vi "TestTracer.vi"() -> ()   [LabVIEW 2018]
uses:
  8343dff0-8b7c-4e66-97a3-4b21e463c662.vi
  7eb2ee23-5221-471e-a6d0-41069041a5d2.vi
  88696aa2-b6d8-4ac2-bba1-d74daa604035.vi
  a57bbf11-b234-4300-b227-3b603d238aca.vi
  ee03f129-e9c8-4ab2-bbd6-a9c7767b6f28.vi
  0673ade5-3870-4221-86d1-9f763805091c.vi
  TracerLibrary/Tracer/protected/SendMessage.vi
  TracerLibrary/Tracer/protected/Timestamp.vi
  TracerLibrary/Tracer/Tracer_Level-Debug.vi
  TracerLibrary/Tracer/protected/Tracer_ClassAttributes.vi
  TracerLibrary/Tracer/Tracer_Level-Warning.vi
  TracerLibrary/Tracer/Tracer_Level-Info.vi
  TracerLibrary/Tracer/Tracer_Level-Error.vi
  TracerLibrary/Tracer/Tracer.lvclass
panel:
  out "Ms / Tracecall":dbl
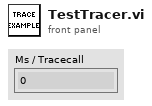
[diagram p1: front panel]
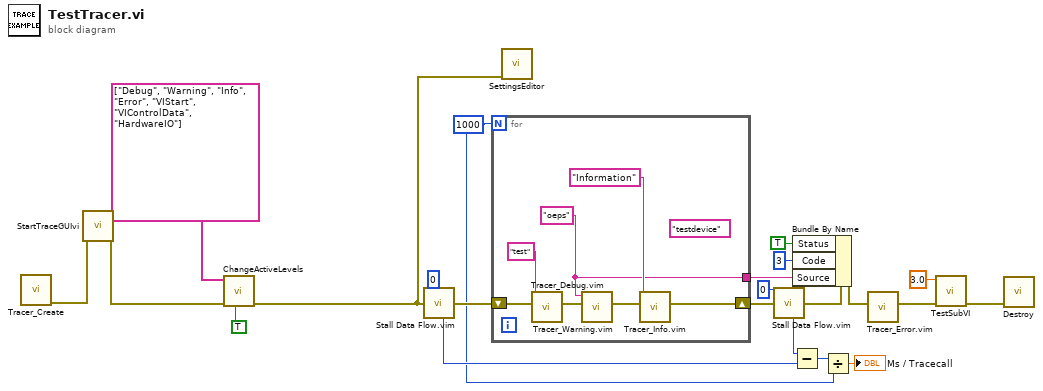
[diagram p0: block diagram]
diagram:
  w5 = 1000
  n1 = call "Tracer_Create.vi"() -> ("Error Out"=w14:errorcluster)  [unwired: 11 in]
  n2 = call "StartTraceGUIvi.vi"("Error In"=w14) -> ("Error Out"=w22:errorcluster)  [unwired: 10 in]
  n3 = call "ChangeActiveLevels.vi"("Force Update"=TRUE ("Force update"), "Error In"=w22, "Active Levels"=string[] ["Debug", "Warning", "Info", "Error", "VIStart", "VIControlData", "HardwareIO"] ("Active Compressed in")) -> ("Error Out"=w16:errorcluster)  [unwired: 8 in]
  n4 = call "Stall Data Flow.vim"("value in"=w16, "milliseconds to wait"=u32 0) -> ("millisecond timer value"=w7:u32, "value out"=w18:errorcluster)
  n5 = for {
    N: w5 -> [_]
    tunnel: [w24] -> w10
    shift-right: [w26] -> w21
    shift-left: w18 -> [w29]
    (unwired) "testdevice" ("Device")
    w24 = "oeps" ("WarningText")
    n6 = call "Tracer_Debug.vim"("Error In"=w29, "Text"="test") -> ("Error Out"=w28:errorcluster)  [unwired: 9 in]
    n7 = call "Tracer_Warning.vim"("Error In"=w28, "Warning Text"=w24) -> ("Error Out"=w27:errorcluster)  [unwired: 9 in]
    n8 = call "Tracer_Info.vim"("Error In"=w27, "Info Text"="Information" ("WarningText")) -> ("Error Out"=w26:errorcluster)  [unwired: 9 in]
  }
  n9 = call "SettingsEditor.vi"("Error In"=w16) -> ()  [unwired: 10 in, 1 out]
  n10 = call "Stall Data Flow.vim"("value in"=w21, "milliseconds to wait"=u32 0) -> ("millisecond timer value"=w8:u32, "value out"=w17:errorcluster)
  n11 = Subtract(x=w8, y=w7) -> (x-y=w6:u32)
  n12 = Bundle By Name(cluster=w17, "Status"=TRUE ("status"), "Code"=3 ("code"), "Source"=w10) -> (w20:errorcluster)
  n13 = Divide(x=w6, y=w5) -> (x/y=→"Ms / Tracecall":dbl)
  n14 = call "Tracer_Error.vim"("Error In"=w20) -> ("Error Out"=w19:errorcluster)  [unwired: 10 in]
  n15 = call "TestSubVI.vi"("Error In"=w19, "Numeric"=3.0) -> ("Error Out"=w15:errorcluster)  [unwired: 9 in]
  n16 = call "Destroy.vi"("Error In"=w15) -> ()  [unwired: 10 in, 1 out]
